vi "Get Display Image.vi"(8 "error in (no error)":errorcluster, 11 "CallVIStep in":refnum<class "CallVIStep.lvclass">) -> (0 "error out":errorcluster, 2 "Image":picture, 3 "CallVIStep out":refnum<class "CallVIStep.lvclass">)   [LabVIEW 2015, in "CallVIStep.lvclass"]
uses:
  CallVIStep.lvclass
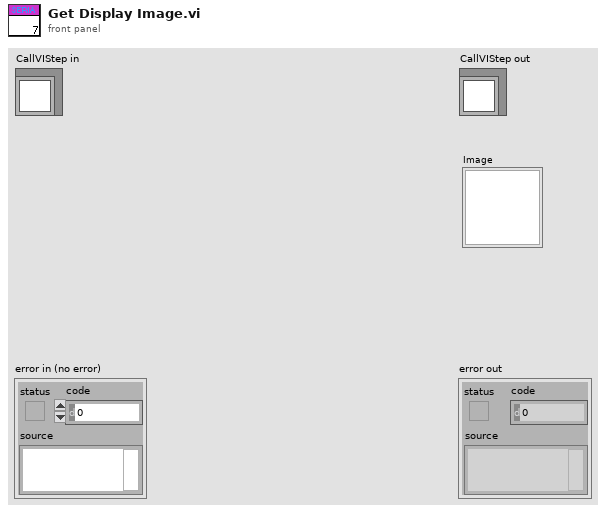
[diagram p1: front panel]
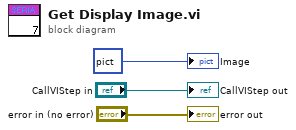
[diagram p0: block diagram]
diagram:
  "error out" <- "error in (no error)"
  "CallVIStep out" <- "CallVIStep in"
  "Image" <- picture bytes[830] ("Image")
